vi "Fire Event item.vi"(8 "error in (no error)":errorcluster, 11 "Event":string[](array[string])) -> (0 "internal error out":errorcluster)   [LabVIEW 2020]
uses:
  Event log.ctl
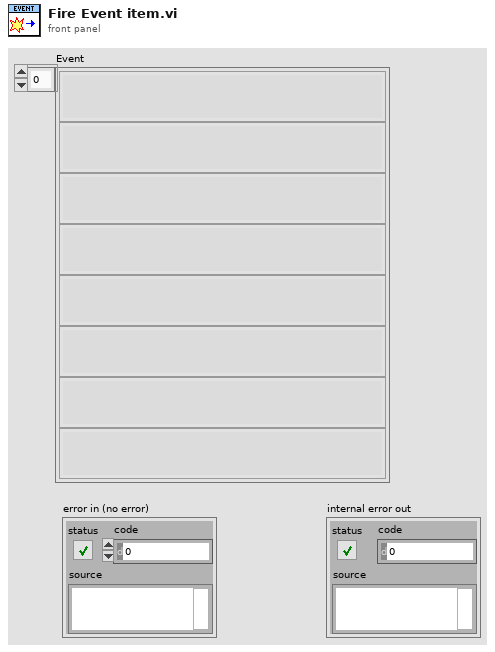
[diagram p1: front panel]
types:
  T1 = typedef "Event log.ctl" = cluster{"Time":timestamp, "Event":string[]}
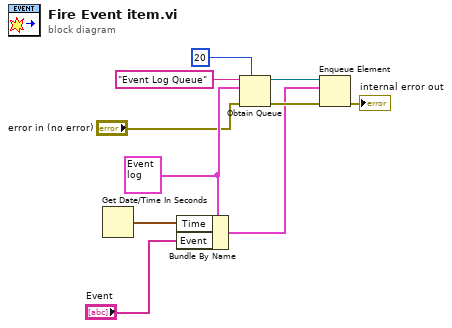
[diagram p0: block diagram]
diagram:
  w5 = T1 {"Time"=timestamp(0 s since 1904-01-01), "Event"=[]}
  n1 = Get Date/Time In Seconds() -> (seconds since 1Jan1904=w4:timestamp)
  n2 = Bundle By Name(cluster=w5, "Time"=w4, "Event"="Event") -> (w1:T1)
  n3 = Obtain Queue(max queue size (-1, unlimited)=20, name (unnamed)="Event Log Queue", element data type=w5, error in (no error)="error in (no error)") -> (queue out=w8:refnum<queue>, error out=w7:errorcluster)  [unwired: 1 in, 1 out]
  n4 = Enqueue Element(queue=w8, element=w1, error in (no error)=w7) -> (error out=→"internal error out":errorcluster)  [unwired: 1 in, 2 out]
